vi "ReadDoorState.vi"(8 "error in (no error)":errorcluster, 11 "reference in":refnum<class "Door.lvclass">) -> (0 "error out":errorcluster, 2 "DoorState":bool, 3 "reference out":refnum<class "Door.lvclass">)   [LabVIEW 2020, in "Door.lvclass"]
uses:
  Door.lvclass
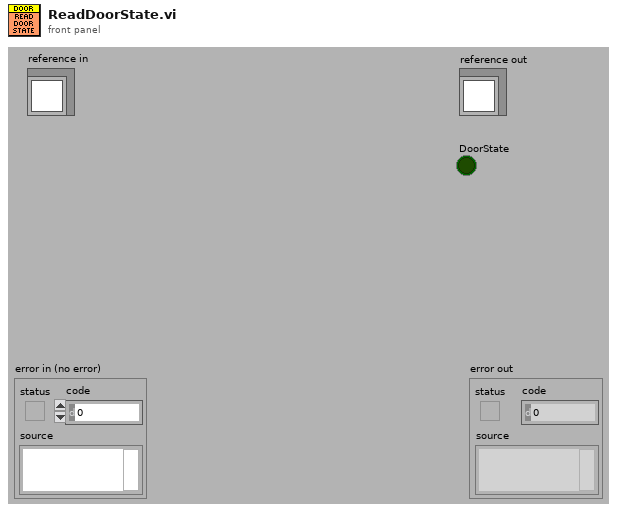
[diagram p1: front panel]
types:
  T1 = typedef "Door.lvclass/ObjectAttributes.ctl" = cluster{"DoorState":bool}
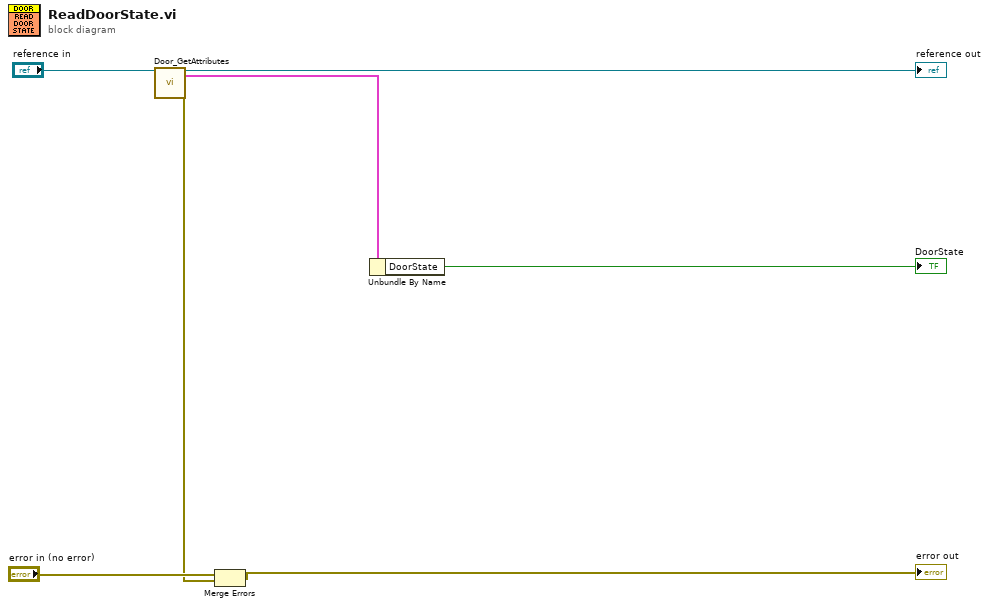
[diagram p0: block diagram]
diagram:
  n1 = call "Door_GetAttributes.vi"("reference in"="reference in") -> ("reference out"=→"reference out":refnum<class "Door.lvclass">, "Data"=w4:T1, "error out"=w2:errorcluster)  [unwired: 15 in, 1 out]
  n2 = Merge Errors("error in (no error)", w2) -> (→"error out":errorcluster)
  n3 = Unbundle By Name(w4) -> ("DoorState"=→"DoorState":bool)
